vi "open excel get worksheet names.vi"(8 "error in (no error)":errorcluster, 10 "milliseconds to wait":u32, 11 "report file path":path) -> (0 "error out":errorcluster, 1 "Number of Sample Sheets":i32, 2 "worksheets count":i32, 3 "NI_report out":refnum<class "NI_report.lvclass">, 4 "start of Sample Sheets":i32, 5 "Worksheet Names":string[](array[string]))   [LabVIEW 2016]
uses:
  <vilib>/Utility/NIReport.llb/NI_report.lvclass
  <vilib>/addons/_office/NI_ReportGenerationToolkit.lvlib
  <vilib>/Utility/NIReport.llb/Excel/NI_Excel.lvclass
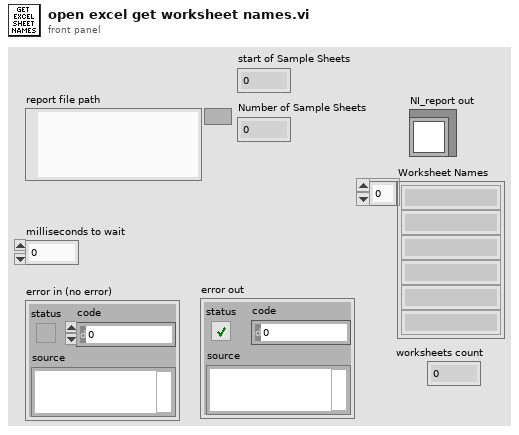
[diagram p1: front panel]
types:
  T1 = enum16{"maximized", "minimized", "normal", "no change"}
  T2 = enum16{"Standard Report", "HTML", "Word", "Excel"}
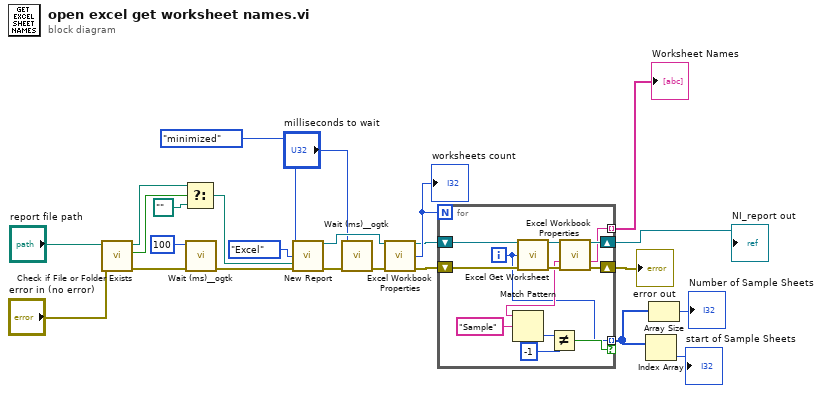
[diagram p0: block diagram]
diagram:
  n1 = call <vilib>:"Check if File or Folder Exists.vi"("error in (no error)"="error in (no error)", "path"="report file path") -> ("error out"=w8:errorcluster, "file or folder exists?"=w9:bool, "dup path"=w10:path)  [unwired: 7 in]
  n2 = Select(t=w10, s=w9, f=path "") -> (s? t:f=w11:path)
  n3 = call "Wait (ms)__ogtk.vi"("error in (no error)"=w8, "milliseconds to wait"=u32 100) -> ("error out"=w16:errorcluster)  [unwired: 8 in, 1 out]
  n4 = call <vilib>:"New Report.vi"("window state (normal)"=T1."minimized", "report type"=T2."Excel", "template (empty)"=w11, "error in (no error)"=w16) -> ("report out"=w18:refnum<class "NI_report.lvclass">, "error out"=w13:errorcluster)  [unwired: 10 in]
  n5 = call "Wait (ms)__ogtk.vi"("error in (no error)"=w13, "milliseconds to wait"="milliseconds to wait") -> ("error out"=w19:errorcluster)  [unwired: 8 in, 1 out]
  n6 = call <vilib>:"Excel Workbook Properties.vi"("report in"=w18, "error in (no error)"=w19) -> ("report out"=w21:refnum<class "NI_report.lvclass">, "worksheets count"=w22:i32, "error out"=w20:errorcluster)  [unwired: 10 in, 1 out]
  "worksheets count" <- w22
  n7 = for {
    N: w22 -> [_]
    shift-right: [w31] -> w14
    shift-left: w20 -> [w36]
    shift-right: [w32] -> w23
    shift-left: w21 -> [w35]
    tunnel: [w30] -> w24 mode=indexing
    tunnel: [w25] -> w3 mode=indexing if=w26
    i -> [w25]
    n8 = call <vilib>:"Excel Get Worksheet.vi"("report in"=w35, "worksheet index (0)"=w25, "error in (no error)"=w36) -> ("report out"=w33:refnum<class "NI_report.lvclass">, "error out"=w34:errorcluster)  [unwired: 11 in]
    n9 = call <vilib>:"Excel Workbook Properties.vi"("report in"=w33, "error in (no error)"=w34) -> ("report out"=w32:refnum<class "NI_report.lvclass">, "current worksheet name"=w30:string, "error out"=w31:errorcluster)  [unwired: 10 in, 1 out]
    n10 = Match Pattern(string=w30, regular expression="Sample") -> (offset past match=w28:i32)  [unwired: 1 in, 3 out]
    n11 = Not Equal?(x=w28, y=-1) -> (x != y?=w26:bool)
  }
  "Worksheet Names" <- w24
  "NI_report out" <- w23
  "error out" <- w14
  n12 = Index Array(array=w3) -> (element=→"start of Sample Sheets":i32)  [unwired: 1 in]
  n13 = Array Size(array=w3) -> (size(s)=→"Number of Sample Sheets":i32)
